vi "get_voltage_limits.vi"(8 "error in":errorcluster, 11 "PI P123.01 & PiezoDrive TD250 & NI USB 7855R in":refnum<class "PI P123.01 & PiezoDrive TD250 & NI USB 7855R.lvclass">) -> (0 "error out":errorcluster, 1 "Voltage_furthest":i16, 2 "Voltage_closest":i16, 3 "PI P123.01 & PiezoDrive TD250 & NI USB 7855R out":refnum<class "PI P123.01 & PiezoDrive TD250 & NI USB 7855R.lvclass">)   [LabVIEW 2020, in "PI P123.01 & PiezoDrive TD250 & NI USB 7855R.lvclass"]
uses:
  PI P123.01 & PiezoDrive TD250 & NI USB 7855R.lvclass
  PI P123.01 & PiezoDrive TD250 & NI USB 7855R.lvclass/PI P123.01 & PiezoDrive TD250 & NI USB 7855R.ctl
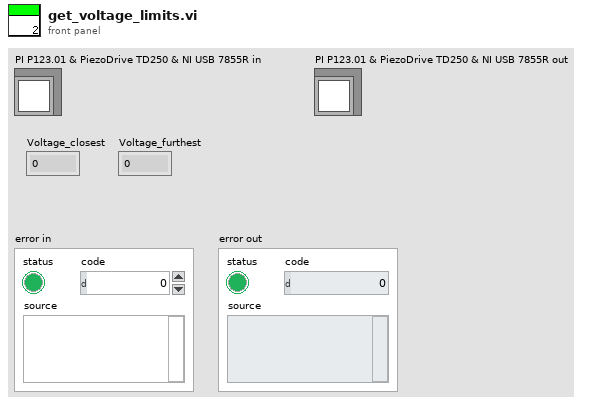
[diagram p1: front panel]
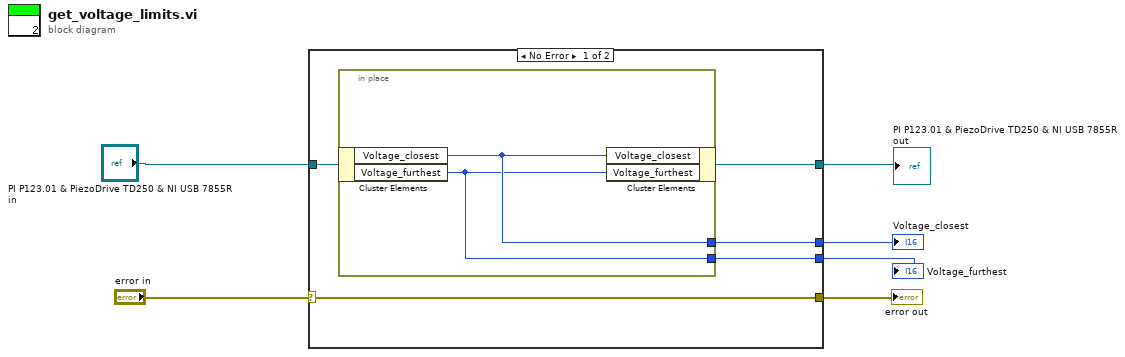
[diagram p0: block diagram]
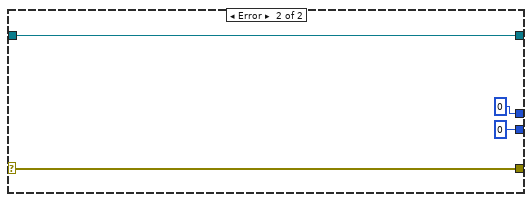
[diagram p2: hidden frame]
diagram:
  n1 = case shown="No Error" "error in" {
    selector: "error in" -> [w9 w16]
    tunnel: "PI P123.01 & PiezoDrive TD250 & NI USB 7855R in" -> [w11 w17]
    tunnel: [w10 w17] -> w5
    tunnel: [w9 w16] -> w3
    tunnel: [w8 i16 0 ("Piezo_maximum")] -> w2
    tunnel: [w7 i16 0 ("Piezo_minimum")] -> w1
    frame No Error {
      n2 = in-place {
        in-place-border: [w13] -> w8
        in-place-border: [w12] -> w7
        n3 = in-place-cluster #1(w11) -> ("Voltage_closest"=w13:i16, "Voltage_furthest"=w12:i16)
        n4 = in-place-cluster #1("Voltage_closest"=w13, "Voltage_furthest"=w12) -> (w10:refnum<class "PI P123.01 & PiezoDrive TD250 & NI USB 7855R.lvclass">)
      }
    }
    frame Error {
    }
  }
  "PI P123.01 & PiezoDrive TD250 & NI USB 7855R out" <- w5
  "error out" <- w3
  "Voltage_closest" <- w2
  "Voltage_furthest" <- w1
